vi "Set Self Cmd.vi"(8 "error in (no error)":errorcluster, 10 "cmd":i32, 11 "channel":i32) -> (0 "error out":errorcluster)   [LabVIEW 2021, in "vmmso.lvlib"]
doc: "DLL_API void WINAPI SetSelfCmd(int channel, int cmd);"
uses:
  vmmso.lvlib
  vmmso.dll
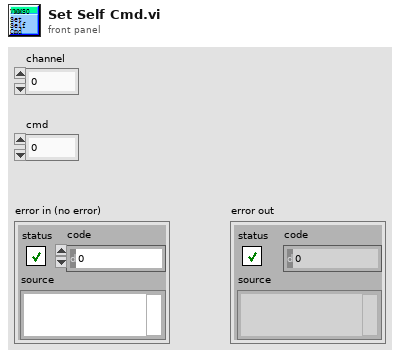
[diagram p1: front panel]
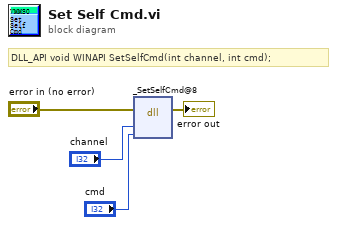
[diagram p0: block diagram]
diagram:
  # "DLL_API void WINAPI SetSelfCmd(int channel, int cmd);"
  n1 = dll-call lib="O:/MSO/library/demo-Labview/vmmso/vmmso.*" fn="_SetSelfCmd@8"(error in="error in (no error)", "channel"="channel", "cmd"="cmd") -> (error out=→"error out":errorcluster)  [unwired: 5 in, 1 out]
